vi "Arrange GObject.vi"(8 "error in (no error)":errorcluster, 10 "Arrange":T1, 11 "GObject in":refnum<vi>) -> (0 "error out":errorcluster, 2 "object arranged?":bool, 3 "GObject out":refnum<vi>)   [LabVIEW 2019, in "Builtins.lvlib"]
doc: "Arranges the selected block diagram objects vertically to align the source terminal to the adjacent sink terminal (left-to-right) or sink to source terminals (right-to-left).\n\nCreated by: Ryan Pacini"
uses:
  Builtins.lvlib
  Arrange.ctl
  Label Position.ctl
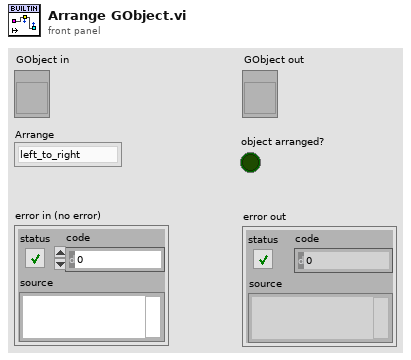
[diagram p1: front panel]
types:
  T1 = typedef "Builtins.lvlib/Arrange.ctl" = enum8{"left_to_right", "right_to_left"}
  T2 = typedef "Builtins.lvlib/Label Position.ctl" = enum8{"Unchanged", "Top-left", "Top-middle", "Top-right", "Right-top", "Right-middle", "Right-bottom", "Bottom-right", "Bottom-middle", "Bottom-left", "Left-bottom", "Left-middle", "Left-top"}
  T3 = typedef "LVRectTypeDef.ctl" = cluster{"Left":i16, "Top":i16, "Right":i16, "Bottom":i16}
  T4 = cluster{"Position":cluster{"h":i16, "v":i16}, "Flags":i32, "Type":enum32{"LooseEnd", "Endpoint", "Bend", "Junction"}, "Up Joint Index":i16, "Down Joint Index":i16, "Left Joint Index":i16, "Right Joint Index":i16}[]
  T5 = typedef "LVPositionTypeDef.ctl" = cluster{"Left":i32, "Top":i32}
  T6 = cluster{"Left":i32, "Top":i32, "Right":i32, "Bottom":i32}
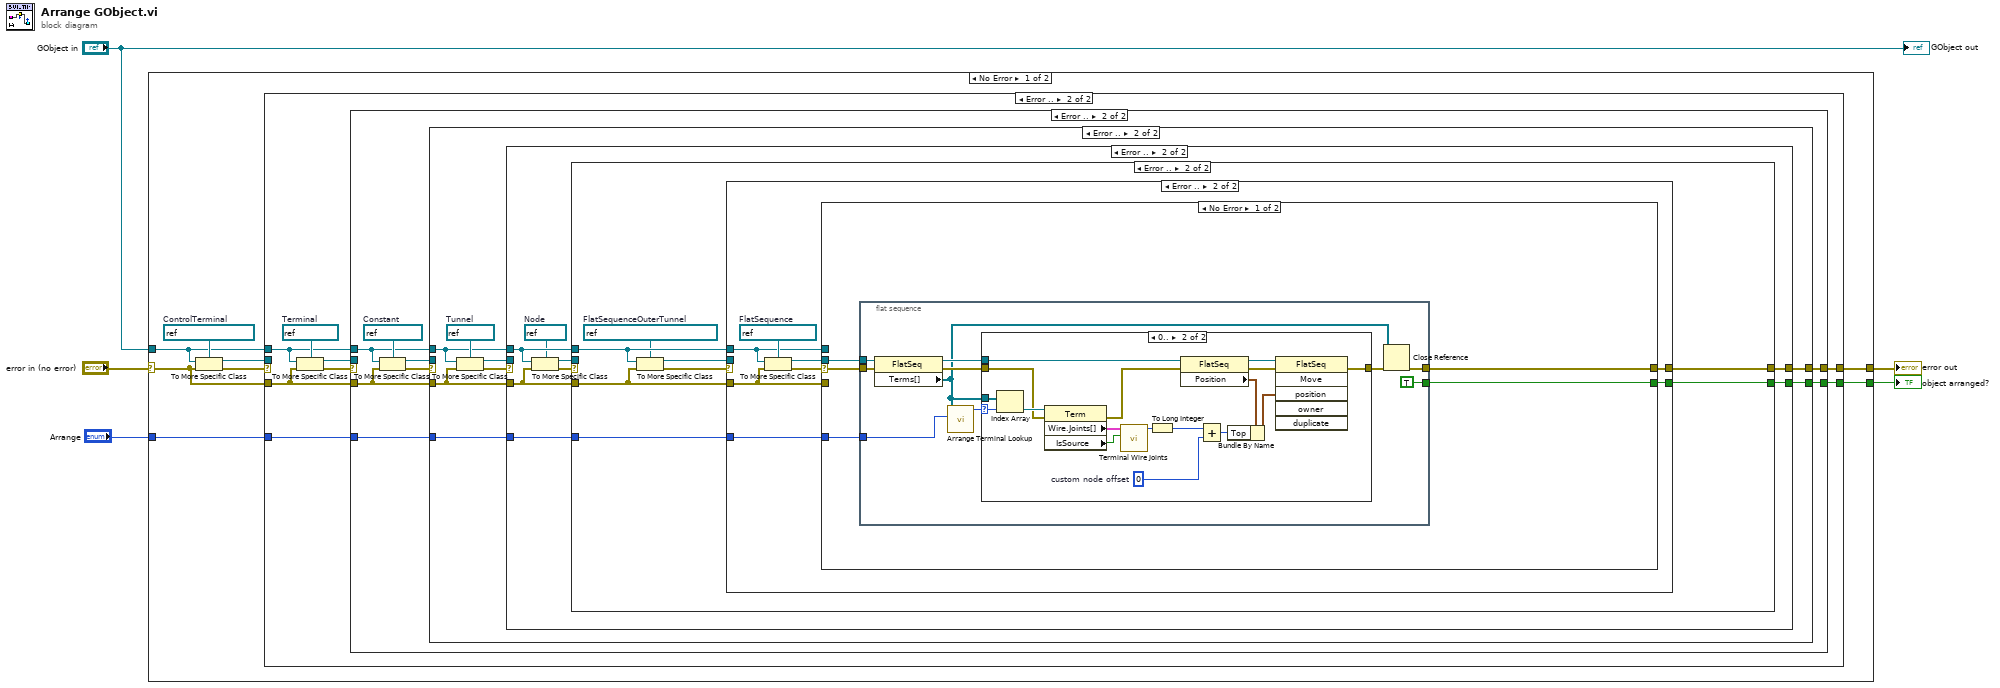
[diagram p0: block diagram]
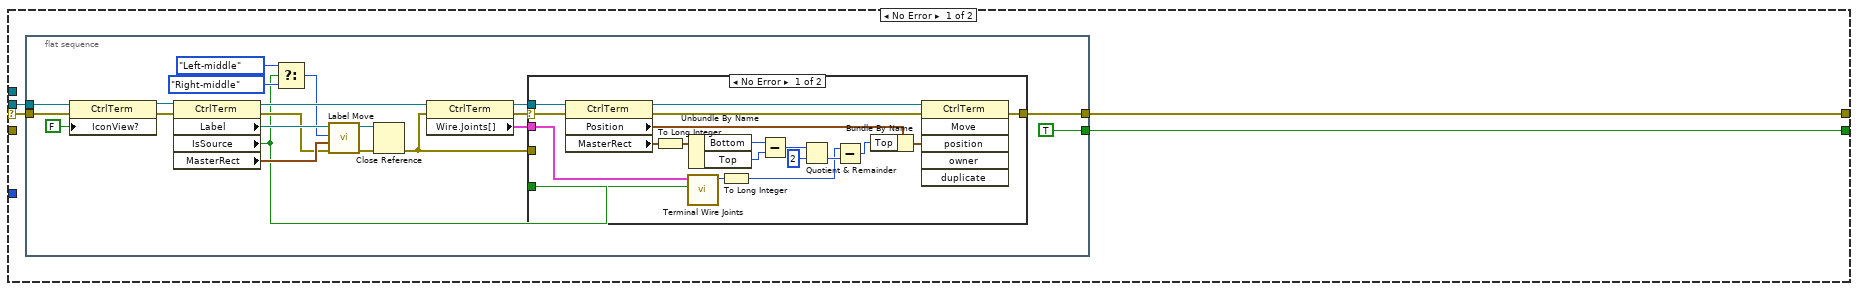
[diagram p2: hidden frame]
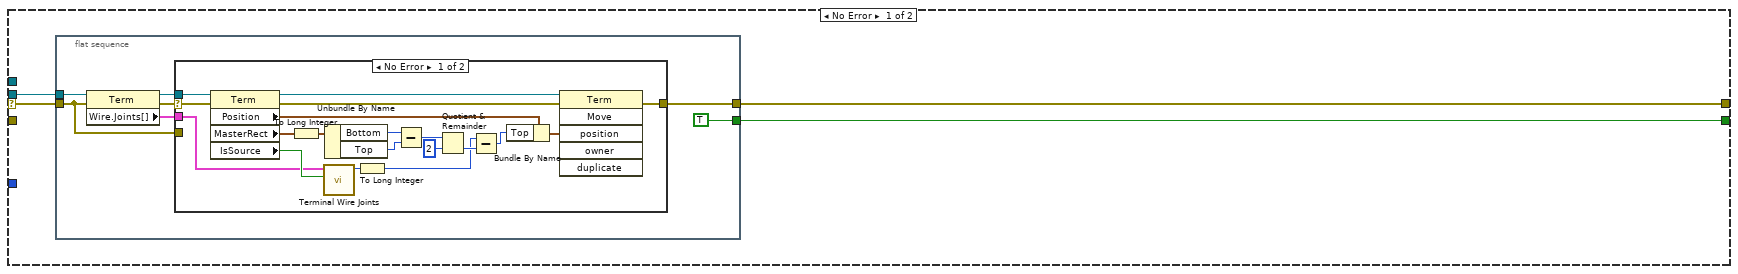
[diagram p4: hidden frame]
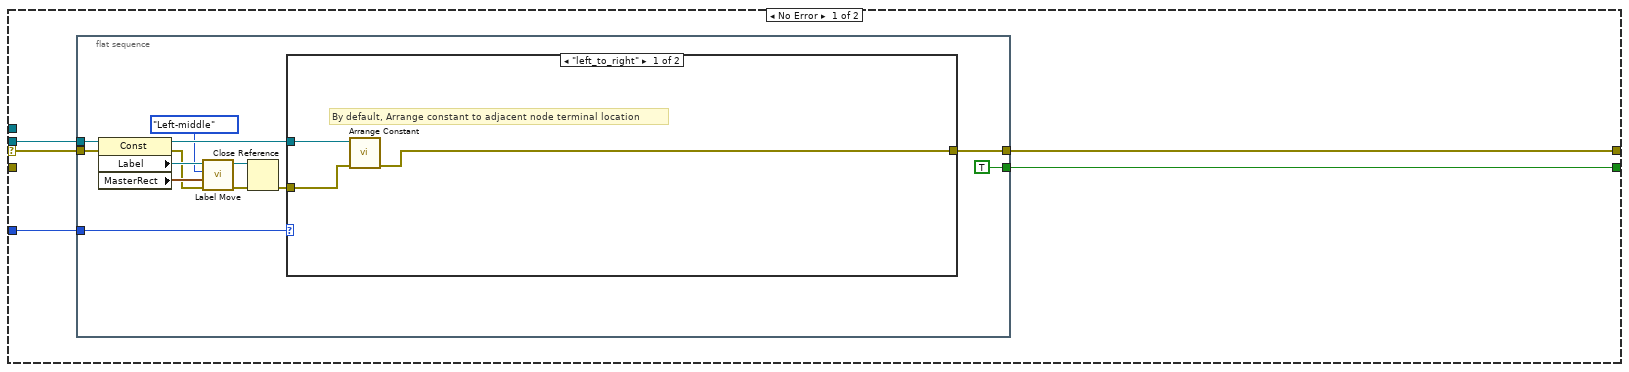
[diagram p6: hidden frame]
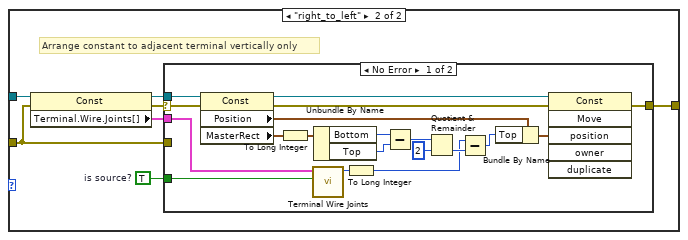
[diagram p7: hidden frame]
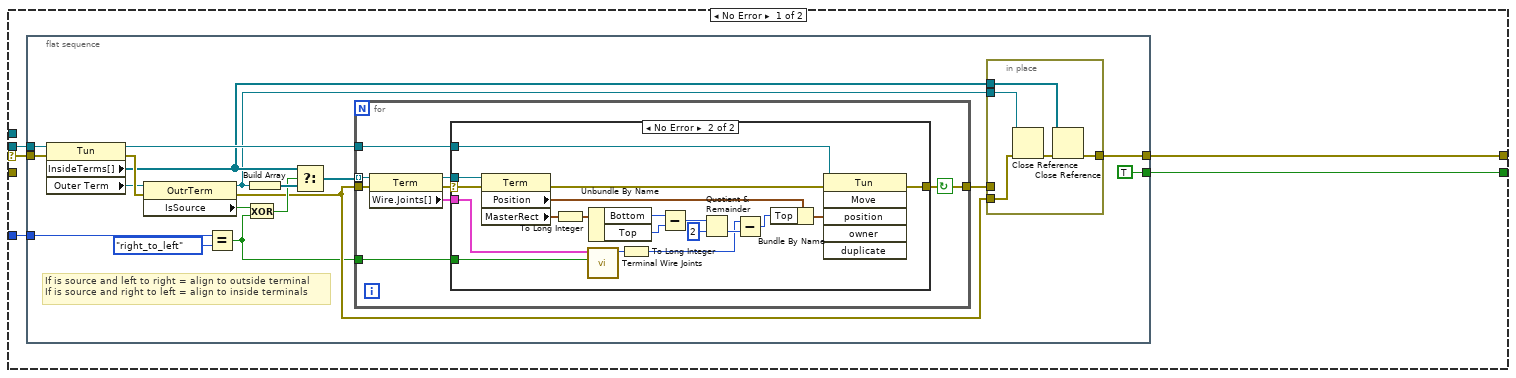
[diagram p9: hidden frame]
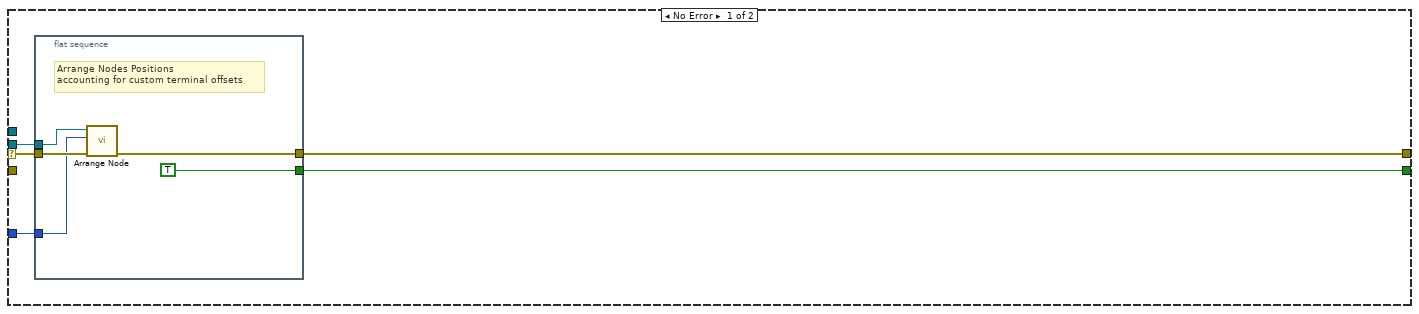
[diagram p11: hidden frame]
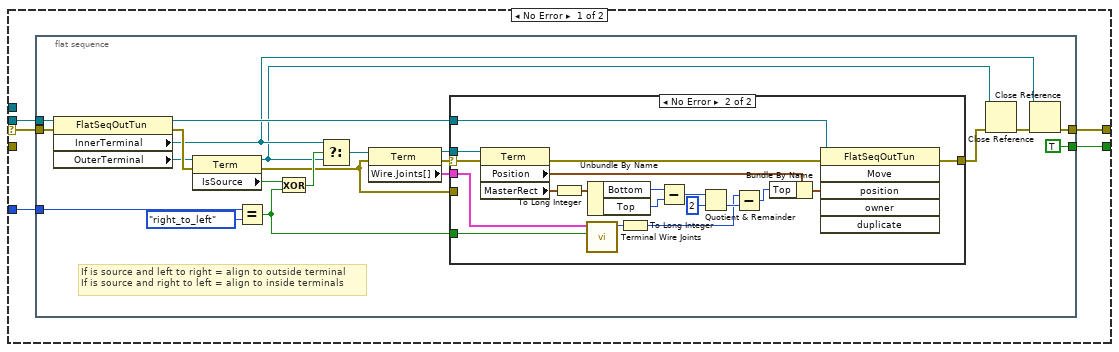
[diagram p12: hidden frame]
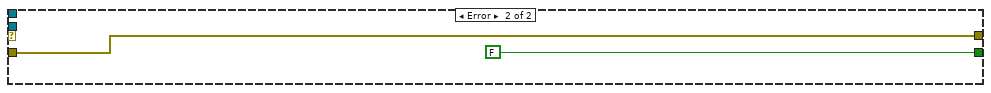
[diagram p15: hidden frame]
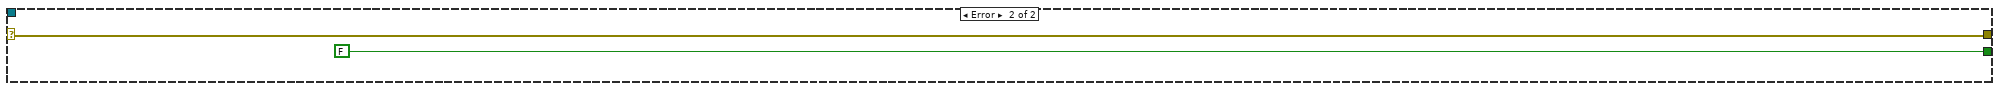
[diagram p16: hidden frame]
diagram:
  n1 = case shown="No Error" "error in (no error)" {
    selector: "error in (no error)" -> [w10 w334]
    tunnel: "GObject in" -> [w9 _]
    tunnel: [w8 w334] -> w3
    tunnel: [w7 FALSE] -> w1
    tunnel: "Arrange" -> [w6 _]
    frame No Error {
      w13 = refnum<vi> refnum  # ControlTerminal
      n2 = To More Specific Class(target class=w13, reference=w9, error in=w10) -> (specific class reference=w11:refnum<vi>, error out=w12:errorcluster)
      n3 = case shown="Error .." w12 {
        selector: w12 -> [w17 _]
        tunnel: w11 -> [w16 _]
        tunnel: [w15 w61] -> w8
        tunnel: w10 -> [_ w63]
        tunnel: w9 -> [_ w62]
        tunnel: w6 -> [_ w60]
        tunnel: [w14 w59] -> w7
        frame No Error {
          n4 = flat-sequence {
            tunnel: w17 -> [w38]
            tunnel: w16 -> [w37]
            tunnel: [w27] -> w15
            tunnel: [TRUE] -> w14
            frame #0 {
              n5 = property class="CtrlTerm"(reference=w37, error in=w38, "IconView?"=FALSE ("Icon View?")) -> (reference out=w34:refnum<vi>, error out=w35:errorcluster)
              n6 = property class="CtrlTerm"(reference=w34, error in=w35) -> (reference out=w28:refnum<vi>, error out=w31:errorcluster, "Label"=w33:refnum<vi>, "IsSource"=w19:bool, "MasterRect"=w32:T3)
              n7 = Select(t=Label_Position."Left-middle" ("Label Position"), s=w19, f=Label_Position."Right-middle" ("Label Position")) -> (s? t:f=w18:T2)
              n8 = call "Label Move.vi"("error in (no error)"=w31, "Owner Master Bounds Rect"=w32, "Label Position"=w18, "Label in"=w33) -> ("error out"=w30:errorcluster, "dup Label"=w29:refnum<vi>)  [unwired: 6 in]
              n9 = Close Reference(reference=w29, error in (no error)=w30) -> (error out=w22:errorcluster)
              n10 = property class="CtrlTerm"(reference=w28, error in=w22) -> (reference out=w25:refnum<vi>, error out=w24:errorcluster, "Wire.Joints[]"=w23:T4)
              n11 = case shown="No Error" w24 {
                selector: w24 -> [w40 _]
                tunnel: w19 -> [w45 _]
                tunnel: [w42 w58] -> w27
                tunnel: w25 -> [w41 _]
                tunnel: w23 -> [w39 _]
                tunnel: w22 -> [_ w58]
                frame No Error {
                  n12 = property class="CtrlTerm"(reference=w41, error in=w40) -> (reference out=w57:refnum<vi>, error out=w56:errorcluster, "Position"=w55:T5, "MasterRect"=w53:T3)
                  n13 = To Long Integer(number=w53) -> (32bit integer=w50:T6)
                  n14 = call "Terminal Wire Joints.vi"("Is Source?"=w45, "Joints"=w39) -> ("Vertical Position"=w44:i16)  [unwired: 8 in, 1 out]
                  n15 = Unbundle By Name(w50) -> ("Bottom"=w52:i32, "Top"=w51:i32)
                  n16 = To Long Integer(number=w44) -> (32bit integer=w43:i32)
                  n17 = Subtract(x=w52, y=w51) -> (x-y=w49:i32)
                  n18 = Quotient & Remainder(x=w49, y=2) -> (floor(x/y)=w47:i32)  [unwired: 1 out]
                  n19 = Subtract(x=w43, y=w47) -> (x-y=w46:i32)
                  n20 = Bundle By Name(cluster=w55, "Top"=w46) -> (w54:T5)
                  n21 = invoke class="CtrlTerm" method="Move"(reference=w57, error in=w56, "position"=w54) -> (error out=w42:errorcluster)  [unwired: 3 in, 5 out]
                }
                frame Error {
                }
              }
            }
          }
        }
        frame Error {
          w66 = refnum<vi> refnum  # Terminal
          n22 = To More Specific Class(target class=w66, reference=w62, error in=w63) -> (specific class reference=w64:refnum<vi>, error out=w65:errorcluster)
          n23 = case shown="Error .." w65 {
            selector: w65 -> [w70 _]
            tunnel: w64 -> [w69 _]
            tunnel: w63 -> [_ w101]
            tunnel: w62 -> [_ w102]
            tunnel: [w68 w100] -> w61
            tunnel: w60 -> [_ w99]
            tunnel: [w67 w98] -> w59
            frame No Error {
              n24 = flat-sequence {
                tunnel: w70 -> [w71]
                tunnel: w69 -> [w76]
                tunnel: [w77] -> w68
                tunnel: [TRUE] -> w67
                frame #0 {
                  n25 = property class="Term"(reference=w76, error in=w71) -> (reference out=w74:refnum<vi>, error out=w73:errorcluster, "Wire.Joints[]"=w72:T4)
                  n26 = case shown="No Error" w73 {
                    selector: w73 -> [w79 _]
                    tunnel: [w82 w97] -> w77
                    tunnel: w74 -> [w80 _]
                    tunnel: w72 -> [w78 _]
                    tunnel: w71 -> [_ w97]
                    frame No Error {
                      n27 = property class="Term"(reference=w80, error in=w79) -> (reference out=w96:refnum<vi>, error out=w95:errorcluster, "Position"=w94:T5, "MasterRect"=w92:T3, "IsSource"=w81:bool)
                      n28 = To Long Integer(number=w92) -> (32bit integer=w89:T6)
                      n29 = call "Terminal Wire Joints.vi"("Is Source?"=w81, "Joints"=w78) -> ("Vertical Position"=w84:i16)  [unwired: 8 in, 1 out]
                      n30 = Unbundle By Name(w89) -> ("Bottom"=w91:i32, "Top"=w90:i32)
                      n31 = To Long Integer(number=w84) -> (32bit integer=w83:i32)
                      n32 = Subtract(x=w91, y=w90) -> (x-y=w88:i32)
                      n33 = Quotient & Remainder(x=w88, y=2) -> (floor(x/y)=w86:i32)  [unwired: 1 out]
                      n34 = Subtract(x=w83, y=w86) -> (x-y=w85:i32)
                      n35 = Bundle By Name(cluster=w94, "Top"=w85) -> (w93:T5)
                      n36 = invoke class="Term" method="Move"(reference=w96, error in=w95, "position"=w93) -> (error out=w82:errorcluster)  [unwired: 3 in, 5 out]
                    }
                    frame Error {
                    }
                  }
                }
              }
            }
            frame Error {
              w105 = refnum<vi> refnum  # Constant
              n37 = To More Specific Class(target class=w105, reference=w102, error in=w101) -> (specific class reference=w103:refnum<vi>, error out=w104:errorcluster)
              n38 = case shown="Error .." w104 {
                selector: w104 -> [w110 _]
                tunnel: w103 -> [w109 _]
                tunnel: w102 -> [_ w157]
                tunnel: w101 -> [_ w158]
                tunnel: [w108 w155] -> w100
                tunnel: w99 -> [w106 w156]
                tunnel: [w107 w154] -> w98
                frame No Error {
                  n39 = flat-sequence {
                    tunnel: w110 -> [w116]
                    tunnel: w109 -> [w117]
                    tunnel: [w118] -> w108
                    tunnel: [TRUE] -> w107
                    tunnel: w106 -> [w111]
                    frame #0 {
                      n40 = property class="Const"(reference=w117, error in=w116) -> (reference out=w114:refnum<vi>, error out=w121:errorcluster, "Label"=w123:refnum<vi>, "MasterRect"=w122:T3)
                      n41 = call "Label Move.vi"("error in (no error)"=w121, "Owner Master Bounds Rect"=w122, "Label Position"=Label_Position."Left-middle", "Label in"=w123) -> ("error out"=w120:errorcluster, "dup Label"=w119:refnum<vi>)  [unwired: 6 in]
                      n42 = Close Reference(reference=w119, error in (no error)=w120) -> (error out=w113:errorcluster)
                      n43 = case shown="\"left_to_right\"" w111 {
                        tunnel: [w124 w133] -> w118
                        tunnel: w114 -> [w125 w132]
                        tunnel: w113 -> [w126 w131]
                        frame "left_to_right" {
                          # "By default, Arrange constant to adjacent node terminal location"
                          n44 = call "Arrange Constant.vi"("error in (no error)"=w126, "GObject in"=w125) -> ("error out"=w124:errorcluster)  [unwired: 7 in, 2 out]
                        }
                        frame "right_to_left" {
                          w130 = TRUE  # is source?
                          # "Arrange constant to adjacent terminal vertically only"
                          n45 = property class="Const"(reference=w132, error in=w131) -> (reference out=w129:refnum<vi>, error out=w127:errorcluster, "Terminal.Wire.Joints[]"=w128:T4)
                          n46 = case shown="No Error" w127 {
                            selector: w127 -> [w134 _]
                            tunnel: [w138 w153] -> w133
                            tunnel: w130 -> [w137 _]
                            tunnel: w129 -> [w136 _]
                            tunnel: w128 -> [w135 _]
                            tunnel: w131 -> [_ w153]
                            frame No Error {
                              n47 = property class="Const"(reference=w136, error in=w134) -> (reference out=w152:refnum<vi>, error out=w151:errorcluster, "Position"=w150:T5, "MasterRect"=w148:T3)
                              n48 = To Long Integer(number=w148) -> (32bit integer=w145:T6)
                              n49 = call "Terminal Wire Joints.vi"("Is Source?"=w137, "Joints"=w135) -> ("Vertical Position"=w140:i16)  [unwired: 8 in, 1 out]
                              n50 = Unbundle By Name(w145) -> ("Bottom"=w147:i32, "Top"=w146:i32)
                              n51 = To Long Integer(number=w140) -> (32bit integer=w139:i32)
                              n52 = Subtract(x=w147, y=w146) -> (x-y=w144:i32)
                              n53 = Quotient & Remainder(x=w144, y=2) -> (floor(x/y)=w142:i32)  [unwired: 1 out]
                              n54 = Subtract(x=w139, y=w142) -> (x-y=w141:i32)
                              n55 = Bundle By Name(cluster=w150, "Top"=w141) -> (w149:T5)
                              n56 = invoke class="Const" method="Move"(reference=w152, error in=w151, "position"=w149) -> (error out=w138:errorcluster)  [unwired: 3 in, 5 out]
                            }
                            frame Error {
                            }
                          }
                        }
                      }
                    }
                  }
                }
                frame Error {
                  w161 = refnum<vi> refnum  # Tunnel
                  n57 = To More Specific Class(target class=w161, reference=w157, error in=w158) -> (specific class reference=w159:refnum<vi>, error out=w160:errorcluster)
                  n58 = case shown="Error .." w160 {
                    selector: w160 -> [w166 _]
                    tunnel: w159 -> [w165 _]
                    tunnel: w158 -> [_ w222]
                    tunnel: w157 -> [_ w223]
                    tunnel: w156 -> [w164 w221]
                    tunnel: [w163 w220] -> w155
                    tunnel: [w162 w219] -> w154
                    frame No Error {
                      n59 = flat-sequence {
                        tunnel: w166 -> [w184]
                        tunnel: w165 -> [w183]
                        tunnel: w164 -> [w169]
                        tunnel: [w173] -> w163
                        tunnel: [TRUE] -> w162
                        frame #0 {
                          # "If is source and left to right = align to outside terminal\nIf is source and right to left = align to inside terminals"
                          n60 = property class="Tun"(reference=w183, error in=w184) -> (reference out=w176:refnum<vi>, error out=w182:errorcluster, "InsideTerms[]"=w175:refnum<vi>[], "Outer Term"=w181:refnum<vi>)
                          n61 = property class="OutrTerm"(reference=w181, error in=w182) -> (reference out=w174:refnum<vi>, error out=w171:errorcluster, "IsSource"=w179:bool)
                          n62 = Equal?(x=w169, y=Arrange."right_to_left" ("Arrange")) -> (x = y?=w167:bool)
                          n63 = Exclusive Or(1:w167, 2:w179) -> (0:w178:bool)
                          n64 = Build Array(w174) -> (w180:refnum<vi>[])
                          n65 = Select(t=w175, s=w178, f=w180) -> (s? t:f=w177:refnum<vi>[])
                          n66 = for {
                            tunnel: w177 -> [w197] mode=indexing
                            tunnel: w167 -> [w195]
                            tunnel: w171 -> [w194]
                            tunnel: w176 -> [w193]
                            tunnel: [w190] -> w172
                            stop <- w190 continue-if-true
                            n67 = property class="Term"(reference=w197, error in=w194) -> (reference out=w191:refnum<vi>, error out=w196:errorcluster, "Wire.Joints[]"=w192:T4)
                            n68 = case shown="No Error" w196 {
                              selector: w196 -> [w198 w204]
                              tunnel: w195 -> [_ w205]
                              tunnel: [w198 w202] -> w190
                              tunnel: w193 -> [_ w201]
                              tunnel: w192 -> [_ w199]
                              tunnel: w191 -> [_ w200]
                              frame Error {
                              }
                              frame No Error {
                                n69 = property class="Term"(reference=w200, error in=w204) -> (error out=w203:errorcluster, "Position"=w207:T5, "MasterRect"=w208:T3)  [unwired: 1 out]
                                n70 = To Long Integer(number=w208) -> (32bit integer=w215:T6)
                                n71 = call "Terminal Wire Joints.vi"("Is Source?"=w205, "Joints"=w199) -> ("Vertical Position"=w210:i16)  [unwired: 8 in, 1 out]
                                n72 = Unbundle By Name(w215) -> ("Bottom"=w217:i32, "Top"=w216:i32)
                                n73 = To Long Integer(number=w210) -> (32bit integer=w209:i32)
                                n74 = Subtract(x=w217, y=w216) -> (x-y=w214:i32)
                                n75 = Quotient & Remainder(x=w214, y=2) -> (floor(x/y)=w212:i32)  [unwired: 1 out]
                                n76 = Subtract(x=w209, y=w212) -> (x-y=w211:i32)
                                n77 = Bundle By Name(cluster=w207, "Top"=w211) -> (w206:T5)
                                n78 = invoke class="Tun" method="Move"(reference=w201, error in=w203, "position"=w206) -> (error out=w202:errorcluster)  [unwired: 3 in, 5 out]
                              }
                            }
                          }
                          n79 = in-place {
                            in-place-border: w175 -> [w189]
                            in-place-border: w172 -> [_]
                            in-place-border: w174 -> [w187]
                            in-place-border: [w186] -> w173
                            in-place-border: w171 -> [w185]
                            n80 = Close Reference(reference=w187, error in (no error)=w185) -> (error out=w188:errorcluster)
                            n81 = Close Reference(reference=w189, error in (no error)=w188) -> (error out=w186:errorcluster)
                          }
                        }
                      }
                    }
                    frame Error {
                      w218 = refnum<vi> refnum  # Node
                      n82 = To More Specific Class(target class=w218, reference=w223, error in=w222) -> (specific class reference=w224:refnum<vi>, error out=w225:errorcluster)
                      n83 = case shown="Error .." w225 {
                        selector: w225 -> [w230 _]
                        tunnel: w224 -> [w229 _]
                        tunnel: w223 -> [_ w241]
                        tunnel: w222 -> [_ w240]
                        tunnel: w221 -> [w228 w237]
                        tunnel: [w227 w239] -> w220
                        tunnel: [w226 w238] -> w219
                        frame No Error {
                          n84 = flat-sequence {
                            tunnel: [TRUE] -> w226
                            tunnel: w229 -> [w233]
                            tunnel: w230 -> [w234]
                            tunnel: w228 -> [w232]
                            tunnel: [w231] -> w227
                            frame #0 {
                              # "Arrange Nodes Positions\naccounting for custom terminal offsets"
                              n85 = call "Arrange Node.vi"("error in (no error)"=w234, "Arrange"=w232, "Node in"=w233) -> ("error out"=w231:errorcluster)  [unwired: 7 in, 1 out]
                            }
                          }
                        }
                        frame Error {
                          w236 = refnum<vi> refnum  # FlatSequenceOuterTunnel
                          n86 = To More Specific Class(target class=w236, reference=w241, error in=w240) -> (specific class reference=w242:refnum<vi>, error out=w243:errorcluster)
                          n87 = case shown="Error .." w243 {
                            selector: w243 -> [w246 _]
                            tunnel: w242 -> [w245 _]
                            tunnel: w241 -> [_ w294]
                            tunnel: w240 -> [_ w295]
                            tunnel: [w247 w292] -> w239
                            tunnel: [w248 w291] -> w238
                            tunnel: w237 -> [w244 w290]
                            frame No Error {
                              n88 = flat-sequence {
                                tunnel: w246 -> [w269]
                                tunnel: w245 -> [w268]
                                tunnel: w244 -> [w262]
                                tunnel: [w257] -> w247
                                tunnel: [TRUE] -> w248
                                frame #0 {
                                # "If is source and left to right = align to outside terminal\nIf is source and right to left = align to inside terminals"
                                n89 = property class="FlatSeqOutTun"(reference=w268, error in=w269) -> (reference out=w261:refnum<vi>, error out=w267:errorcluster, "InnerTerminal"=w260:refnum<vi>, "OuterTerminal"=w266:refnum<vi>)
                                n90 = property class="Term"(reference=w266, error in=w267) -> (reference out=w253:refnum<vi>, error out=w252:errorcluster, "IsSource"=w265:bool)
                                n91 = Equal?(x=w262, y=Arrange."right_to_left" ("Arrange")) -> (x = y?=w249:bool)
                                n92 = Exclusive Or(1:w249, 2:w265) -> (0:w264:bool)
                                n93 = Select(t=w260, s=w264, f=w253) -> (s? t:f=w263:refnum<vi>)
                                n94 = property class="Term"(reference=w263, error in=w252) -> (reference out=w254:refnum<vi>, error out=w256:errorcluster, "Wire.Joints[]"=w255:T4)
                                n95 = case shown="No Error" w256 {
                                selector: w256 -> [_ w276]
                                tunnel: w249 -> [_ w277]
                                tunnel: [w270 w274] -> w259
                                tunnel: w261 -> [_ w273]
                                tunnel: w255 -> [_ w271]
                                tunnel: w254 -> [_ w272]
                                tunnel: w252 -> [w270 _]
                                frame Error {
                                }
                                frame No Error {
                                n96 = property class="Term"(reference=w272, error in=w276) -> (error out=w275:errorcluster, "Position"=w279:T5, "MasterRect"=w280:T3)  [unwired: 1 out]
                                n97 = To Long Integer(number=w280) -> (32bit integer=w287:T6)
                                n98 = call "Terminal Wire Joints.vi"("Is Source?"=w277, "Joints"=w271) -> ("Vertical Position"=w282:i16)  [unwired: 8 in, 1 out]
                                n99 = Unbundle By Name(w287) -> ("Bottom"=w289:i32, "Top"=w288:i32)
                                n100 = To Long Integer(number=w282) -> (32bit integer=w281:i32)
                                n101 = Subtract(x=w289, y=w288) -> (x-y=w286:i32)
                                n102 = Quotient & Remainder(x=w286, y=2) -> (floor(x/y)=w284:i32)  [unwired: 1 out]
                                n103 = Subtract(x=w281, y=w284) -> (x-y=w283:i32)
                                n104 = Bundle By Name(cluster=w279, "Top"=w283) -> (w278:T5)
                                n105 = invoke class="FlatSeqOutTun" method="Move"(reference=w273, error in=w275, "position"=w278) -> (error out=w274:errorcluster)  [unwired: 3 in, 5 out]
                                }
                                }
                                n106 = Close Reference(reference=w253, error in (no error)=w259) -> (error out=w258:errorcluster)
                                n107 = Close Reference(reference=w260, error in (no error)=w258) -> (error out=w257:errorcluster)
                                }
                              }
                            }
                            frame Error {
                              w297 = refnum<vi> refnum  # FlatSequence
                              n108 = To More Specific Class(target class=w297, reference=w294, error in=w295) -> (specific class reference=w293:refnum<vi>, error out=w296:errorcluster)
                              n109 = case shown="No Error" w296 {
                                selector: w296 -> [w302 _]
                                tunnel: w295 -> [_ w332]
                                tunnel: w294 -> [_ _]
                                tunnel: w293 -> [w301 _]
                                tunnel: [w298 w332] -> w292
                                tunnel: [w299 FALSE] -> w291
                                tunnel: w290 -> [w300 _]
                                frame No Error {
                                n110 = flat-sequence {
                                tunnel: [TRUE] -> w299
                                tunnel: w301 -> [w311]
                                tunnel: w302 -> [w309]
                                tunnel: w300 -> [w306]
                                tunnel: [w304] -> w298
                                frame #0 {
                                n111 = property class="FlatSeq"(reference=w311, error in=w309) -> (reference out=w310:refnum<vi>, error out=w308:errorcluster, "Terms[]"=w303:refnum<vi>[])
                                n112 = call "Arrange Terminal Lookup.vi"("Arrange"=w306, "Terminals"=w303) -> ("Terminal Index"=w307:i32)  [unwired: 9 in]
                                n113 = case shown="0.." w307 {
                                selector: w307 -> [_ w318]
                                tunnel: [w313 w330] -> w305
                                tunnel: w310 -> [_ w325]
                                tunnel: w308 -> [w313 w314]
                                tunnel: w303 -> [_ w319]
                                frame ..-1 {
                                }
                                frame 0.. {
                                w317 = 0  # custom node offset
                                n114 = Index Array(array=w319, index=w318) -> (element=w316:refnum<vi>)
                                n115 = property class="Term"(reference=w316, error in=w314) -> (error out=w315:errorcluster, "Wire.Joints[]"=w321:T4, "IsSource"=w320:bool)  [unwired: 1 out]
                                n116 = call "Terminal Wire Joints.vi"("Is Source?"=w320, "Joints"=w321) -> ("Vertical Position"=w324:i16)  [unwired: 8 in, 1 out]
                                n117 = To Long Integer(number=w324) -> (32bit integer=w322:i32)
                                n118 = property class="FlatSeq"(reference=w325, error in=w315) -> (reference out=w328:refnum<vi>, error out=w329:errorcluster, "Position"=w327:T5)
                                n119 = Add(x=w322, y=w317) -> (x+y=w323:i32)
                                n120 = Bundle By Name(cluster=w327, "Top"=w323) -> (w326:T5)
                                n121 = invoke class="FlatSeq" method="Move"(reference=w328, error in=w329, "position"=w326) -> (error out=w330:errorcluster)  [unwired: 3 in, 5 out]
                                }
                                }
                                n122 = Close Reference(reference=w303, error in (no error)=w305) -> (error out=w304:errorcluster)
                                }
                                }
                                }
                                frame Error {
                                }
                              }
                            }
                          }
                        }
                      }
                    }
                  }
                }
              }
            }
          }
        }
      }
    }
    frame Error {
    }
  }
  "error out" <- w3
  "object arranged?" <- w1
  "GObject out" <- "GObject in"
